vi "ObjectHandler.SendExit.vi"(8 "ErrorIn":errorcluster) -> (0 "ErrorOut":errorcluster)   [LabVIEW 2016, in "ObjectHandler.lvclass"]
uses:
  ObjectHandler.lvclass
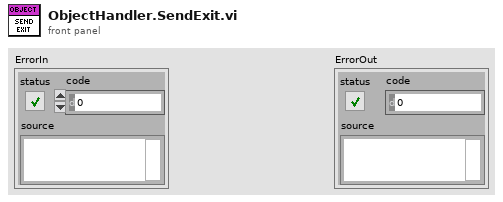
[diagram p1: front panel]
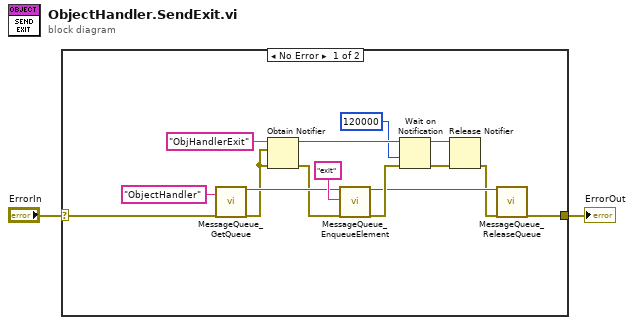
[diagram p0: block diagram]
diagram:
  n1 = case shown="No Error" "ErrorIn" {
    selector: "ErrorIn" -> [w14 w18]
    tunnel: [w3 w18] -> w2
    frame No Error {
      n2 = call "MessageQueue_GetQueue.vi"("Name"="ObjectHandler", "ErrorIn"=w14) -> ("QueueOut"=w15:refnum<queue>, "ErrorOut"=w4:errorcluster)  [unwired: 15 in, 1 out]
      n3 = Obtain Notifier(name (unnamed)="ObjHandlerExit", notification data type=w4, error in (no error)=w4) -> (notifier out=w12:refnum<notifier>, error out=w10:errorcluster)  [unwired: 1 in, 1 out]
      n4 = call "MessageQueue_EnqueueElement.vi"("QueueIn"=w15, "Message"="exit", "ErrorIn"=w10) -> ("QueueOut"=w7:refnum<queue>, "ErrorOut"=w9:errorcluster)  [unwired: 15 in]
      n5 = Wait on Notification(notifier=w12, timeout in ms (-1)=120000, error in (no error)=w9) -> (notifier out=w11:refnum<notifier>, error out=w8:errorcluster)  [unwired: 1 in, 2 out]
      n6 = Release Notifier(notifier=w11, error in (no error)=w8) -> (error out=w6:errorcluster)  [unwired: 1 in, 2 out]
      n7 = call "MessageQueue_ReleaseQueue.vi"("QueueIn"=w7, "ErrorIn"=w6) -> ("ErrorOut"=w3:errorcluster)  [unwired: 15 in, 2 out]
    }
    frame Error {
    }
  }
  "ErrorOut" <- w2
